vi "Create Instrument.vi"(8 "error in (no error)":errorcluster, 9 "Config Path":path, 10 "Subsystem Name":string, 11 "Instrument in":refnum<class "Instrument.lvclass">) -> (0 "error out":errorcluster, 3 "Instrument out":refnum<class "Instrument.lvclass">)   [LabVIEW 2016, in "Instrument.lvclass"]
uses:
  Instrument.lvclass
  C:/Program Files (x86)/National Instruments/LabVIEW 2016/vi.lib/JKI/JKI SMO/SMO/SMO.lvclass
  Typedefs/Configuration--Cluster.ctl
  Configuration/Configuration.lvclass
  Instrument.lvclass/Instrument.ctl
  <vilib>/JKI/JKI SMO/SMO/SMO.lvclass
  Example Instrument/Example Instrument.lvclass
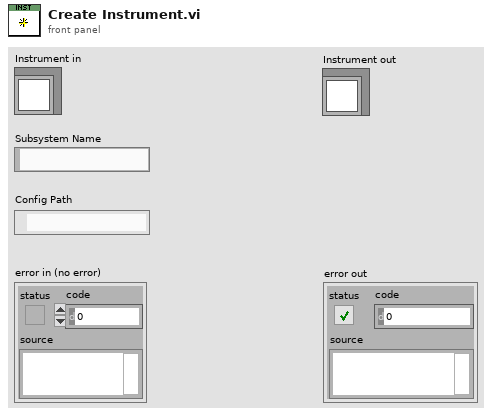
[diagram p1: front panel]
types:
  T1 = typedef "Example Instrument.lvclass/Configuration--Cluster.ctl" = cluster{"VI Address":string, "Hardware Address":string}
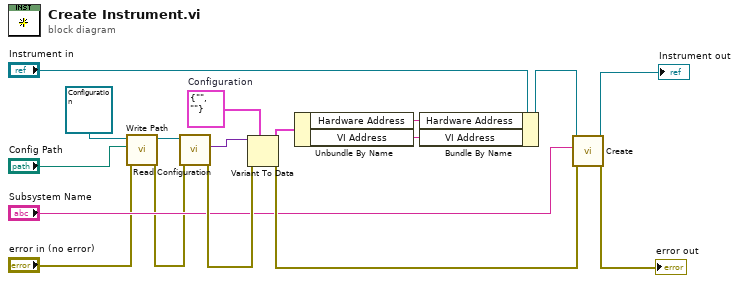
[diagram p0: block diagram]
diagram:
  w13 = T1 {"VI Address"="", "Hardware Address"=""}  # Configuration
  n1 = call-dynamic "Write Path.vi"("error in (no error)"="error in (no error)", "Path"="Config Path", "Configuration in"=refnum<class "Configuration.lvclass"> refnum) -> ("error out"=w3:errorcluster, "Configuration out"=w5:refnum<class "Configuration.lvclass">)  [unwired: 7 in]
  n2 = call "Read Configuration.vi"("error in (no error)"=w3, "Configuration in"=w5) -> ("error out"=w11:errorcluster, "Configuration"=w12:variant)  [unwired: 7 in, 1 out]
  n3 = Variant To Data(error in=w11, type=w13, Variant=w12) -> (data=w1:T1, error out=w15:errorcluster)
  n4 = Unbundle By Name(w1) -> ("Hardware Address"=w16:string, "VI Address"=w17:string)
  n5 = Bundle By Name(cluster="Instrument in", "Hardware Address"=w16, "VI Address"=w17) -> (w8:refnum<class "Instrument.lvclass">)
  n6 = call <vilib>:"Create.vi"("error in (no error)"=w15, "Subsystem Name (optional)"="Subsystem Name", "SMO"=w8) -> ("error out"=→"error out":errorcluster, "SMO out"=→"Instrument out":refnum<class "Instrument.lvclass">)  [unwired: 6 in, 1 out]
